vi "Test Lockin API.vi"() -> ()   [LabVIEW 2019]
uses:
  src/Instrument.Lockin/Instrument.Lockin.lvclass
  src/Instrument.DAQ/Typedefs/DAQ.Configuration--Cluster--Array.ctl
  src/Instrument.DAQ/Typedefs/DAQ.Configuration--Cluster.ctl
  src/Instrument.DAQ/Typedefs/DAQ.Config.AO.Range--enum.ctl
  src/Instrument.DAQ/Typedefs/DAQ.Config.AI.Range--enum.ctl
  src/Instrument.DAQ/Typedefs/DAQ.Config.AI.Coupling--enum.ctl
  src/Instrument.DAQ/Typedefs/DAQ.TerminalConfiguration--ring.ctl
  <vilib>/addons/_JKI Toolkits/Caraya/classes/Test Suite/Define Test Suite (Default).vi
  <vilib>/addons/_JKI Toolkits/Caraya/classes/Test Suite/Test Suite.lvclass
  src/Instrument.DAQ/Instrument.DAQ.lvclass
panel:
  out "Instrument.Lockin out":refnum<class "Instrument.Lockin.lvclass">
  in  "Instrument.Lockin in":refnum<class "Instrument.Lockin.lvclass">
  # "NOTE:\nBefore running make sure that \"Same f\" = FALSE"
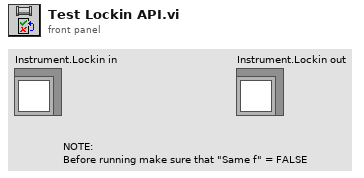
[diagram p1: front panel]
types:
  T1 = typedef "Instrument.Lockin.lvlib/Instrument.DAQ.lvclass/DAQ.Configuration--Cluster--Array.ctl" = T2[]
  T2 = typedef "Instrument.Lockin.lvlib/Instrument.DAQ.lvclass/DAQ.Configuration--Cluster.ctl" = cluster{"Device":string, "AO.Ch":string, "AO.Range":T3, "AI.Ch":string, "AI.Range":T4, "AI.Coupling":T5, "AI terminal config":T6, "AO terminal config":T6}
  T3 = typedef "Instrument.Lockin.lvlib/Instrument.DAQ.lvclass/DAQ.Config.AO.Range--enum.ctl" = enum16{"±0.1", "±1.0", "±10.0", ""}
  T4 = typedef "Instrument.Lockin.lvlib/Instrument.DAQ.lvclass/DAQ.Config.AI.Range--enum.ctl" = enum16{"±0.316", "±1.00", "±3.16", "±10.0", "±31.6", "±42.4", ""}
  T5 = typedef "Instrument.Lockin.lvlib/Instrument.DAQ.lvclass/DAQ.Config.AI.Coupling--enum.ctl" = u16
  T6 = typedef "Instrument.Lockin.lvlib/Instrument.DAQ.lvclass/DAQ.TerminalConfiguration--ring.ctl" = i32
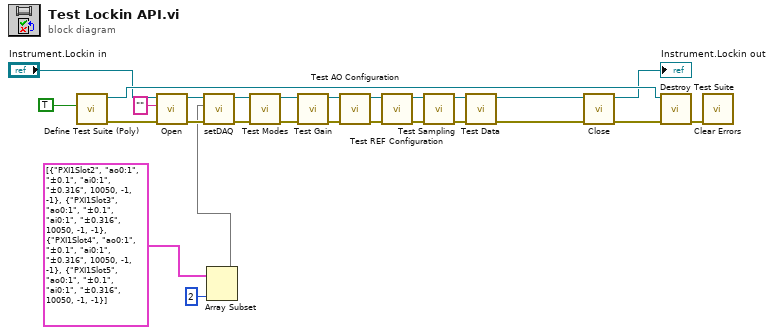
[diagram p0: block diagram]
diagram:
  n1 = call-poly <vilib>:"Define Test Suite (Poly).vi"("Interactive"=TRUE) -> ("error out"=w13:errorcluster, "Test Suite"=w22:refnum<class "Test Suite.lvclass">)  [unwired: 8 in, 1 out]
  n2 = call-dynamic "Open.vi"("error in (no error)"=w13, "address"="" ("Address"), "Instrument.Lockin in"="Instrument.Lockin in") -> ("error out"=w11:errorcluster, "Instrument.Lockin out"=w10:refnum<class "Instrument.Lockin.lvclass">)  [unwired: 7 in]
  n3 = Array Subset(array=T1 [{"Device"="PXI1Slot2", "AO.Ch"="ao0:1", "AO.Range"=enum."±0.1", "AI.Ch"="ai0:1", "AI.Range"=enum."±0.316", "AI.Coupling"=10050, "AI terminal config"=-1, "AO terminal config"=-1}, {"Device"="PXI1Slot3", "AO.Ch"="ao0:1", "AO.Range"=enum."±0.1", "AI.Ch"="ai0:1", "AI.Range"=enum."±0.316", "AI.Coupling"=10050, "AI terminal config"=-1, "AO terminal config"=-1}, {"Device"="PXI1Slot4", "AO.Ch"="ao0:1", "AO.Range"=enum."±0.1", "AI.Ch"="ai0:1", "AI.Range"=enum."±0.316", "AI.Coupling"=10050, "AI terminal config"=-1, "AO terminal config"=-1}, {"Device"="PXI1Slot5", "AO.Ch"="ao0:1", "AO.Range"=enum."±0.1", "AI.Ch"="ai0:1", "AI.Range"=enum."±0.316", "AI.Coupling"=10050, "AI terminal config"=-1, "AO terminal config"=-1}] ("setDAQ"), length=2) -> (w1:T1)  [unwired: 1 in]
  n4 = call-dynamic "setDAQ.vi"("error in (no error)"=w11, "setDAQ"=w1, "Instrument.Lockin in"=w10) -> ("error out"=w8:errorcluster, "Instrument.Lockin out"=w9:refnum<class "Instrument.Lockin.lvclass">)  [unwired: 7 in]
  n5 = call "Test Modes.vi"("error in (no error)"=w8, "Instrument.Lockin in"=w9) -> ("error out"=w21:errorcluster, "Instrument.Lockin out"=w27:refnum<class "Instrument.Lockin.lvclass">)  [unwired: 8 in]
  n6 = call "Test Gain.vi"("error in (no error)"=w21, "Instrument.Lockin in"=w27) -> ("error out"=w20:errorcluster, "Instrument.Lockin out"=w26:refnum<class "Instrument.Lockin.lvclass">)  [unwired: 8 in]
  n7 = call "Test AO Configuration.vi"("error in (no error)"=w20, "Instrument.Lockin in"=w26) -> ("error out"=w19:errorcluster, "Instrument.Lockin out"=w25:refnum<class "Instrument.Lockin.lvclass">)  [unwired: 8 in]
  n8 = call "Test REF Configuration.vi"("error in (no error)"=w19, "Instrument.Lockin in"=w25) -> ("error out"=w18:errorcluster, "Instrument.Lockin out"=w24:refnum<class "Instrument.Lockin.lvclass">)  [unwired: 8 in]
  n9 = call "Test Sampling.vi"("error in (no error)"=w18, "Instrument.Lockin in"=w24) -> ("error out"=w17:errorcluster, "Instrument.Lockin out"=w23:refnum<class "Instrument.Lockin.lvclass">)  [unwired: 8 in]
  n10 = call "Test Data.vi"("error in (no error)"=w17, "Instrument.Lockin in"=w23) -> ("error out"=w6:errorcluster, "Instrument.Lockin out"=w7:refnum<class "Instrument.Lockin.lvclass">)  [unwired: 8 in]
  n11 = call-dynamic "Close.vi"("error in (no error)"=w6, "Instrument.Lockin in"=w7) -> ("error out"=w4:errorcluster, "Instrument.Lockin out"=→"Instrument.Lockin out":refnum<class "Instrument.Lockin.lvclass">)  [unwired: 8 in]
  n12 = call-dynamic "Destroy Test Suite.vi"("error in (no error)"=w4, "Test Suite in"=w22) -> ("error out"=w15:errorcluster)  [unwired: 8 in, 1 out]
  n13 = call <vilib>:"Clear Errors.vi"("error in (no error)"=w15) -> ()  [unwired: 5 in, 2 out]
